vi "Handle DAQ Loose Wires.vi"(10 "Name":string, 11 "Value in":dbl) -> (3 "Value out":dbl)   [LabVIEW 2018, in "DAQ.lvlib"]
uses:
  DAQ.lvlib
  Tag VIs/Tag FGV Operation Enum.ctl
  <vilib>/regexp/Match Regular Expression.xnode
  Shared Variables/Dynamic Shared Variables.lvlib
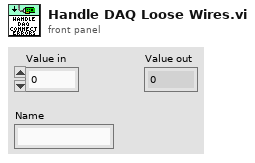
[diagram p1: front panel]
types:
  T1 = typedef "Tag FGV Operation Enum.ctl" = enum16{"Init", "Set Notification Queue", "Create Tag", "Commit", "Write Tag (Numeric)", "Write Tag (Boolean)", "Read All Tags", "Read One Tag", "Delete Tag Category", "Set Alarm Parameters (Numeric)", "Set Alarm Parameters (Boolean)", "Enable All Alarms", "Disable All Alarms", "Delete All Tags", "Read Alarms", "Ack Alarm", "Read Alarm Parameters (Numeric)", "Read Alarm Parameters (Boolean)"}
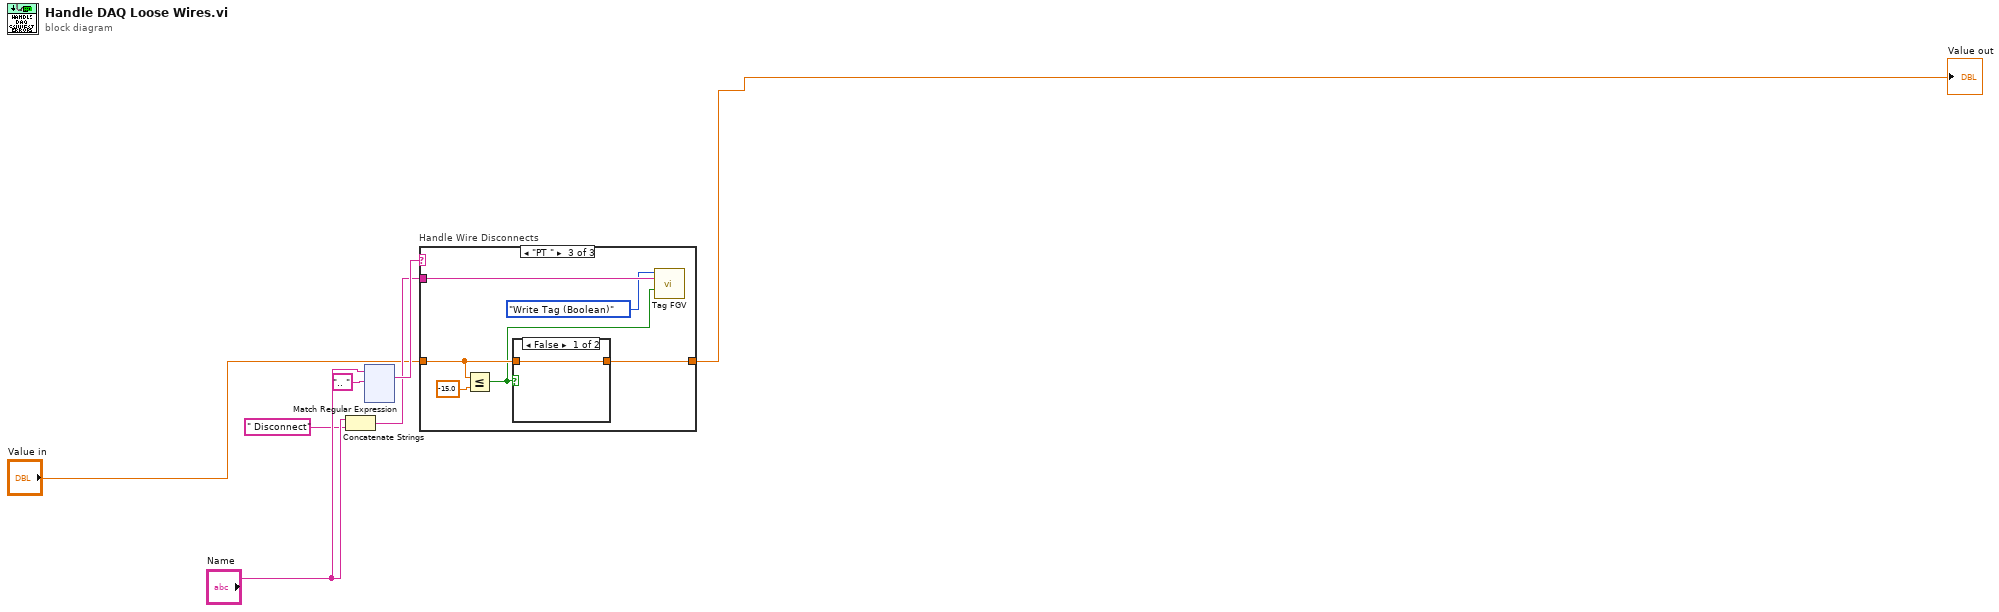
[diagram p0: block diagram]
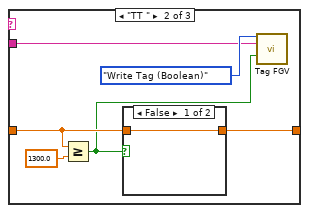
[diagram p3: hidden frame]
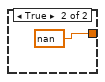
[diagram p4: hidden frame]
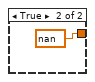
[diagram p5: hidden frame]
diagram:
  n1 = Concatenate Strings("Name", " Disconnect" ("string")) -> (w4:string)
  n2 = xnode "Match Regular Expression"("input string"="Name", "regular expression"=".. ") -> ("whole match"=w5:string)  [unwired: 4 in, 4 out]
  n3 = case "Handle Wire Disconnects" shown="\"PT \"" w5 {
    tunnel: "Value in" -> [w8 w12 w20]
    tunnel: [w8 w13 w21] -> w6
    tunnel: w4 -> [_ w9 w19]
    frame Default {
    }
    frame "TT " {
      n4 = Greater Or Equal?(x=w12, y=1300.0) -> (x >= y?=w10:bool)
      n5 = case shown="False" w10 {
        tunnel: [w15 nan ("mean")] -> w13
        tunnel: w12 -> [w15 _]
        frame False {
        }
        frame True {
        }
      }
      n6 = call "Tag FGV.vi"("Operation"=Tag_FGV_Operation_Enum."Write Tag (Boolean)", "Tag Name"=w9, "Data"=w10) -> ()  [unwired: 5 in, 8 out]
    }
    frame "PT " {
      n7 = Less Or Equal?(x=w20, y=-15.0) -> (x <= y?=w17:bool)
      n8 = case shown="False" w17 {
        tunnel: [w23 nan ("mean")] -> w21
        tunnel: w20 -> [w23 _]
        frame False {
        }
        frame True {
        }
      }
      n9 = call "Tag FGV.vi"("Operation"=Tag_FGV_Operation_Enum."Write Tag (Boolean)", "Tag Name"=w19, "Data"=w17) -> ()  [unwired: 5 in, 8 out]
    }
  }
  "Value out" <- w6
